vi "Status bereits erfasst.vi"(7 "aufsteigend":bool, 8 "error in (no error)":errorcluster caption="Fehler (Eingang, kein Fehler)", 9 "Länge":i32=1, 10 "Status new in":string, 11 "Status old in":string="2024-03-01 Komm Error\n2024-03-01 Druck Error\n2024-03-01 Fluss Error\n2024-03-01 Komm Error\n2024-03-01 Komm Error") -> (0 "error out":errorcluster caption="Fehler (Ausgang)", 1 "unique":bool, 2 "Status new out":string, 3 "Status old out":string)   [LabVIEW 2020, in "Linearisierung v2.lvlib"]
uses:
  Linearisierung v2.lvlib
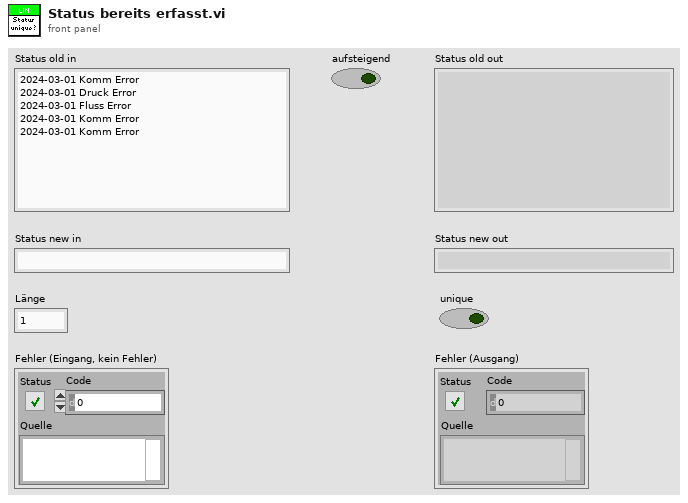
[diagram p1: front panel]
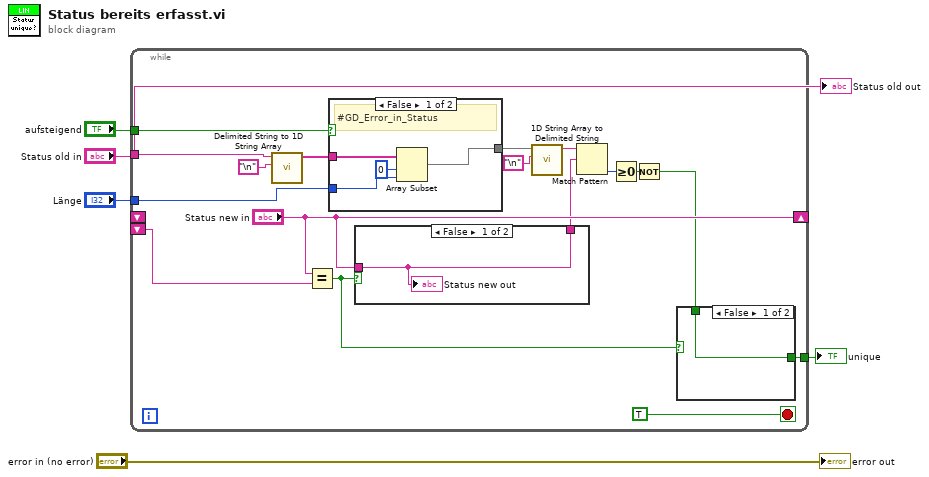
[diagram p0: block diagram]
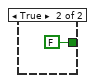
[diagram p2: hidden frame]
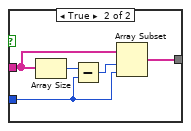
[diagram p4: hidden frame]
diagram:
  n1 = while {
    tunnel: "Status old in" -> [w22]
    tunnel: [w7] -> w3
    tunnel: "aufsteigend" -> [w15]
    tunnel: "Länge" -> [w14]
    shift-right: ["Status new in"] -> _
    shift-left: _ -> [_]
    shift-left: _ -> [w11]
    stop <- TRUE stop-if-true
    n2 = call <vilib>:"Delimited String to 1D String Array.vi"("delimiter"="\n", "delimited string"=w22) -> ("string array"=w21:string[])  [unwired: 9 in]
    n3 = Equal?(x="Status new in", y=w11) -> (x = y?=w8:bool)
    n4 = case shown="False" w15 {
      tunnel: w14 -> [w28 w34]
      tunnel: w21 -> [w29 w31]
      tunnel: [w26 w30] -> w19
      frame False {
        # "#GD_Error_in_Status"
        n5 = Array Subset(array=w29, index=0 ("Index"), length=w28) -> (w26:string[])
      }
      frame True {
        n6 = Array Size(array=w31) -> (size(s)=w33:i32)
        n7 = Subtract(x=w33, y=w34) -> (x-y=w32:i32)
        n8 = Array Subset(array=w31, index=w32, length=w34) -> (w30:string[])
      }
    }
    n9 = case shown="False" w8 {
      tunnel: "Status new in" -> [w25 _]
      tunnel: [w25 _] -> w9
      frame False {
        "Status new out" <- w25
      }
      frame True {
      }
    }
    n10 = call <vilib>:"1D String Array to Delimited String.vi"("delimiter"="\n", "string array"=w19) -> ("delimited string"=w18:string)  [unwired: 9 in]
    n11 = Match Pattern(string=w18, regular expression=w9) -> (offset past match=w17:i32)  [unwired: 1 in, 3 out]
    n12 = Greater Or Equal To 0?(x=w17) -> (x >= 0?=w16:bool)
    n13 = Not(x=w16) -> (.not. x?=w6:bool)
    n14 = case shown="False" w8 {
      tunnel: [w23 FALSE] -> w7
      tunnel: w6 -> [w23 _]
      frame False {
      }
      frame True {
      }
    }
  }
  "unique" <- w3
  "Status old out" <- "Status old in"
  "error out" <- "error in (no error)"
